vi "Set Single Device Microgrid ID.vi"(8 "error in":errorcluster, 10 "DeviceID":T1, 11 "IED in":refnum<class "IED.lvclass">) -> (0 "error out":errorcluster, 3 "IED out":refnum<class "IED.lvclass">)   [LabVIEW 2018, in "IED Actor.lvlib" / "IED.lvclass"]
doc: "Publishes a DDS message to set the MicrogridID of an IED specified by DeviceID."
uses:
  IED.lvclass
  C:/Users/Administrator/Desktop/2018LabVIEW EMS/EMS Generic Actor/EMS Generic/EMS Generic.lvclass
  C:/Users/Administrator/Desktop/2018LabVIEW EMS/IED Actors/Device DDS Communications Framework/Device DDS Communications/Device DDS Communications.lvclass
  <vilib>/ORNL/CSEISMIC DDS/CSEISMIC DDS Base/Data Types/Controls/DeviceID.ctl
  <vilib>/ORNL/CSEISMIC DDS/CSEISMIC DDS Base/Data Types/IED_setMicrogridID.ctl
  Device DDS Communications Framework/Device DDS Communications/Device DDS Communications.lvclass/Device DDS Communications.ctl
  <vilib>/ORNL/CSEISMIC DDS/CSEISMIC DDS Base/CSEISMIC DDS.lvclass/CSEISMIC DDS.ctl
  <vilib>/ORNL/CSEISMIC DDS/CSEISMIC DDS Base/Accessors/Read DDS Reference.vi
  <vilib>/ORNL/CSEISMIC DDS/DDS Writer/DDS Writer.lvclass
  C:/Program Files (x86)/National Instruments/LabVIEW 2018/vi.lib/ORNL/CSEISMIC DDS/CSEISMIC DDS Base/CSEISMIC DDS.lvclass
  <vilib>/ORNL/CSEISMIC DDS/CSEISMIC DDS Base/Error Handler.vi
  Device DDS Communications Framework/Device DDS Communications/Device DDS Communications.lvclass
  <vilib>/ORNL/CSEISMIC DDS/CSEISMIC DDS Base/CSEISMIC DDS.lvclass
  EMS Generic Actor/EMS Generic/EMS Generic.lvclass
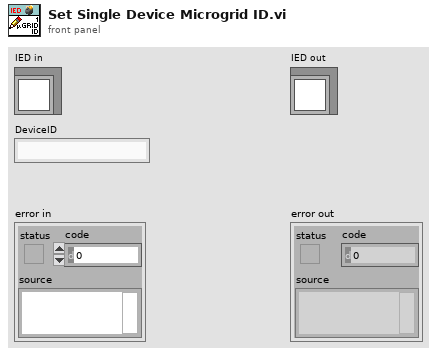
[diagram p1: front panel]
types:
  T1 = typedef "CSEISMIC DDS.lvlib/CSEISMIC DDS.lvclass/DeviceID.ctl" = string
  T2 = typedef "CSEISMIC DDS.lvlib/CSEISMIC DDS.lvclass/IED_setMicrogridID.ctl" = cluster{"DeviceID":T1, "MicrogridID":u8}
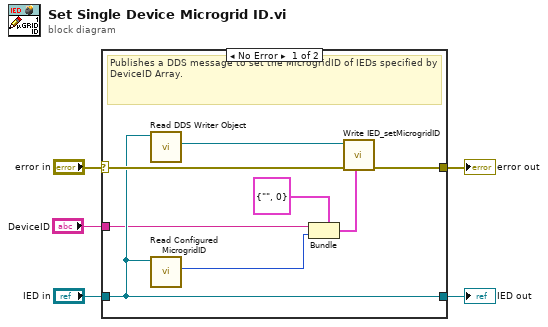
[diagram p0: block diagram]
diagram:
  n1 = case shown="No Error" "error in" {
    selector: "error in" -> [w13 w15]
    tunnel: [w12 w15] -> w4
    tunnel: [w10 w14] -> w2
    tunnel: "IED in" -> [w10 w14]
    tunnel: "DeviceID" -> [w6 _]
    frame No Error {
      # "Publishes a DDS message to set the MicrogridID of IEDs specified by DeviceID Array."
      n2 = call "Read DDS Writer Object.vi"("Device DDS Communications in"=w10) -> ("DDS Writer Object"=w9:refnum<class "DDS Writer.lvclass">)  [unwired: 9 in, 1 out]
      n3 = call "Read Configured MicrogridID.vi"("EMS Generic in"=w10) -> ("Microgrid ID"=w11:u8)  [unwired: 8 in, 2 out]
      n4 = Bundle(cluster=T2 {"DeviceID"="", "MicrogridID"=0} ("Cluster"), "DeviceID"=w6, "MicrogridID"=w11) -> (w7:T2)
      n5 = call <vilib>:"Write IED_setMicrogridID.vi"("IED_setMicrogridID"=w7, "error in"=w13, "DDS Writer in"=w9) -> ("error out"=w12:errorcluster)  [unwired: 7 in, 1 out]
    }
    frame Error {
    }
  }
  "error out" <- w4
  "IED out" <- w2
